vi "myRIO_BRig_Host_v0,20.vi"() -> ()   [LabVIEW 2014]
panel:
  out "output_iTrial":i32
  out "BlockL_T2R_cur":u16 caption="Trials2Reward"
  out "BlockL_BTPR_cur":u16 caption="BadTrialsPostReward"
  out "BlockL_T2R_avg":dbl caption="Trials2Reward" format="%#_3g"
  out "BlockL_BTPR_avg":dbl caption="BadTrialsPostReward" format="%#_3g"
  out "BlockR_T2R_cur":u16 caption="Trials2Reward"
  out "BlockR_BTPR_cur":u16 caption="BadTrialsPostReward"
  out "BlockR_T2R_avg":dbl caption="Trials2Reward" format="%#_3g"
  out "BlockR_BTPR_avg":dbl caption="BadTrialsPostReward" format="%#_3g"
  out "RunTime_minutes":u16
  out "RunTime_seconds":u16
  out "error out 2":errorcluster caption="error out"
  in  "dataIn_maxTrialsDisplayed":u16 caption="Number of Trials Displayed\n( 0 = all trials )"
  in  "colorIn_timeout":u32(colorbox)=7468543 caption="Choice Timeout"
  in  "colorIn_wrong/cue":u32(colorbox)=16728618 caption="Wrong Choice or\nLicked During Cue"
  in  "colorIn_reward":u32(colorbox)=5898088 caption="Reward"
  in  "colorIn_unknown":u32(colorbox)=16449331 caption="Unknown Trial Status"
  in  "LoadPrevSettings":bool
  out "dataOut_plot":cluster{i32[], i32[]}[](graph)
  out "iBlock":u16
  out "iTrial":u16
  in  "stop":bool
  # "Exp Stats"
  # "Current Block Stats"
  # "Trials 2 Reward\n\nBad Trials\nPost Reward"
  # "Left Spout    Right Spout"
  # "Run Time\n\n   minutes    seconds"
  # "Average Block Stats"
  # "Trials 2 Reward\n\nBad Trials\nPost Reward"
  # "Left Spout    Right Spout"
  # "If you get ERROR 5 related to opening a file, press CONTINUE"
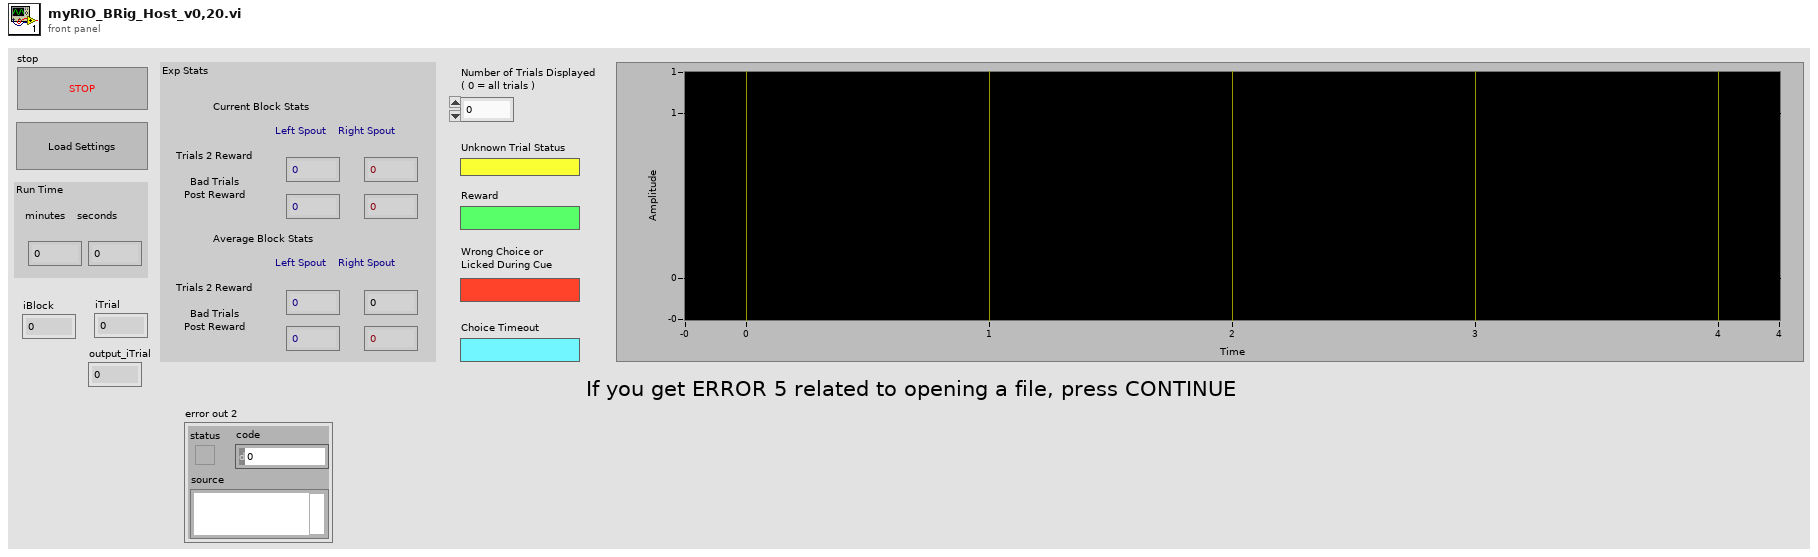
[diagram p1: front panel]
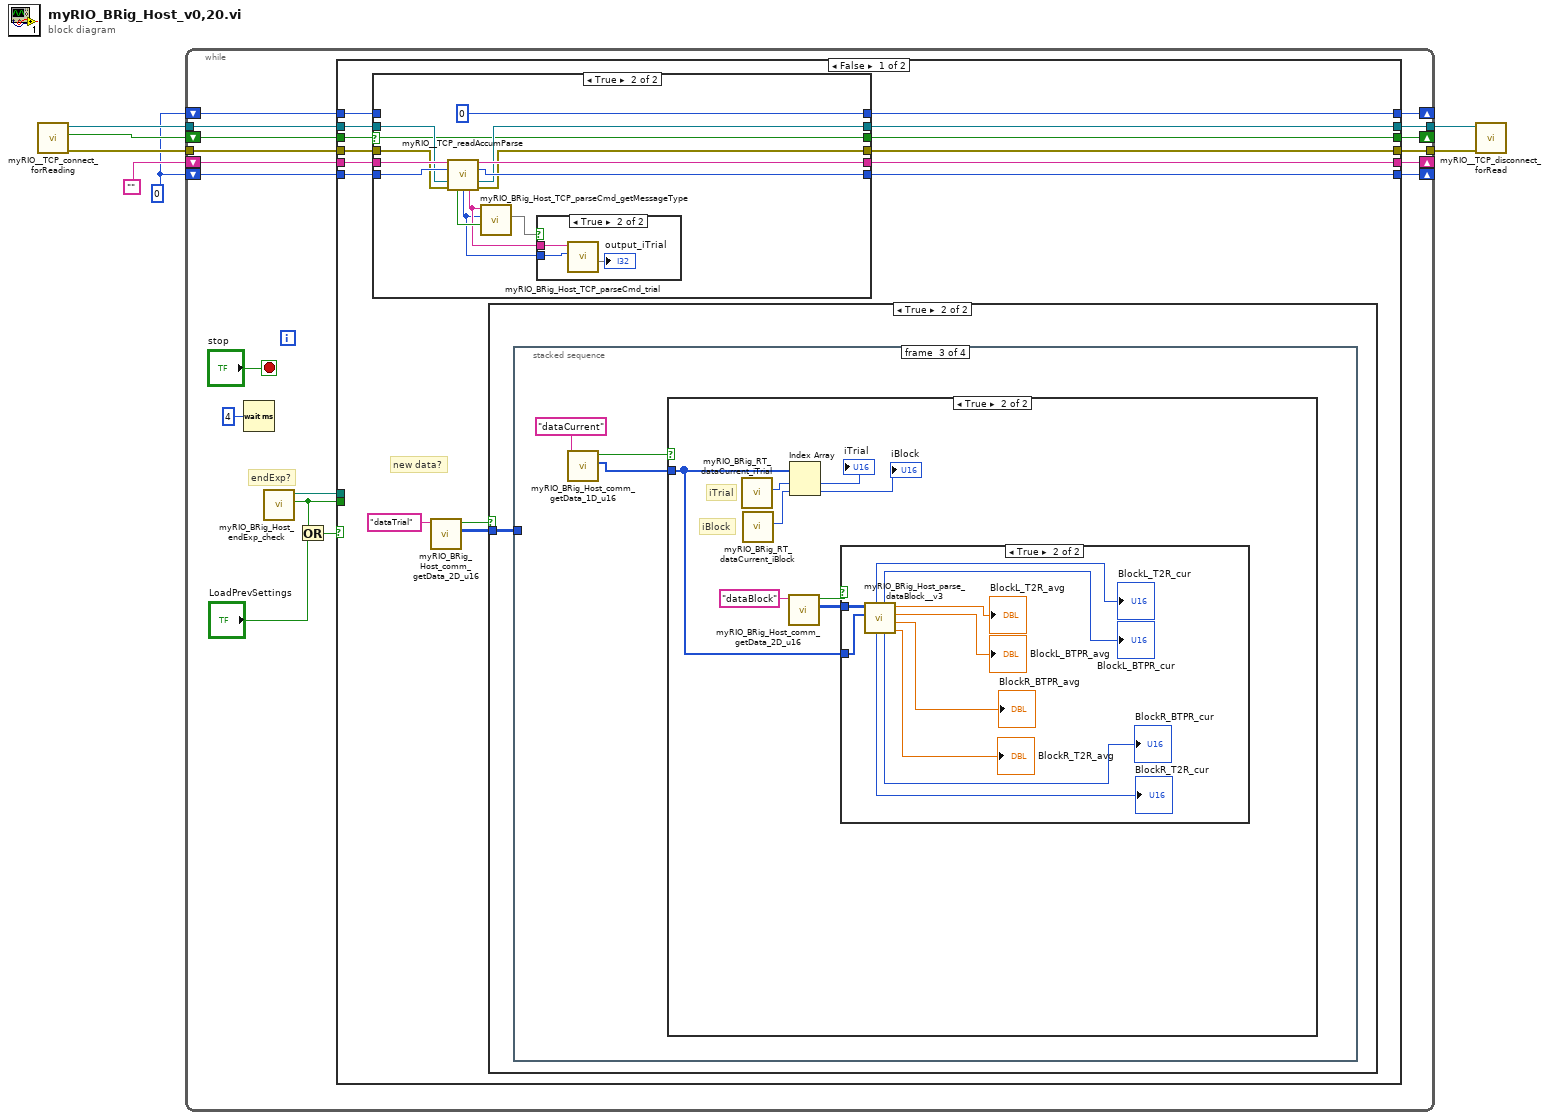
[diagram p0: block diagram]
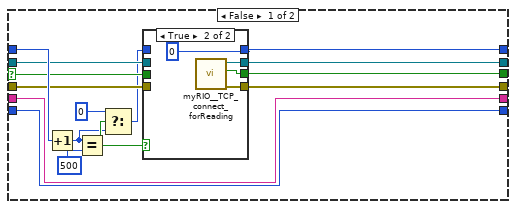
[diagram p2: hidden frame]
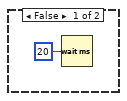
[diagram p5: hidden frame]
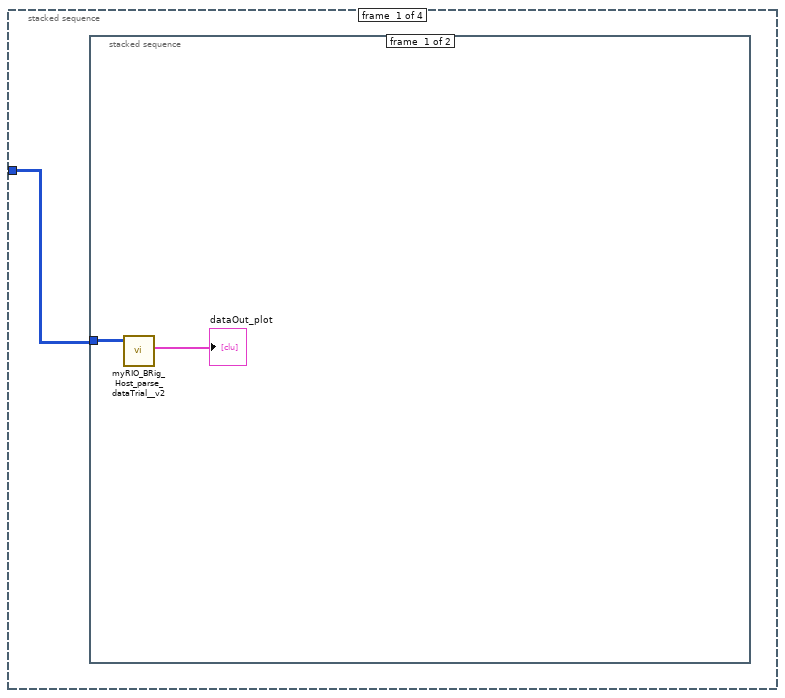
[diagram p6: hidden frame]
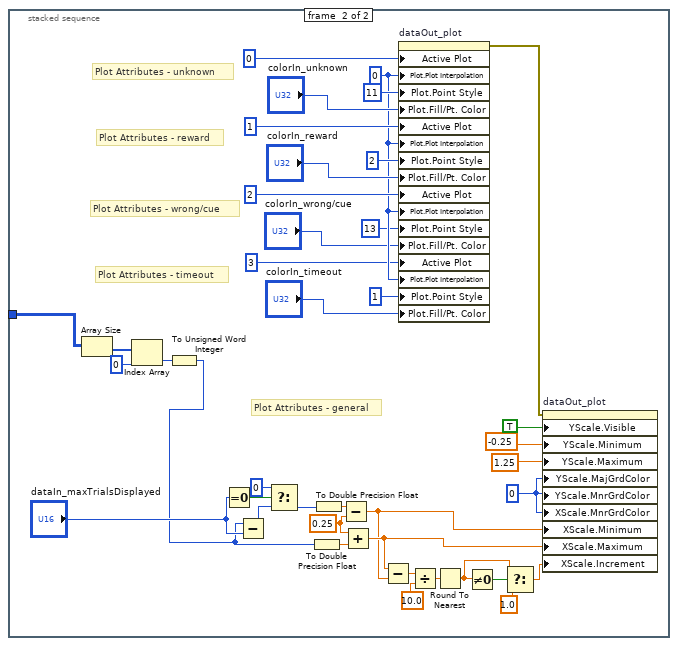
[diagram p7: hidden frame]
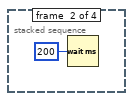
[diagram p8: hidden frame]
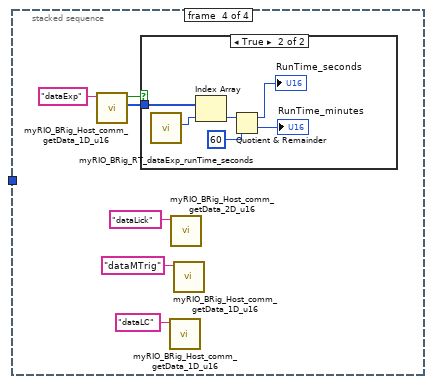
[diagram p11: hidden frame]
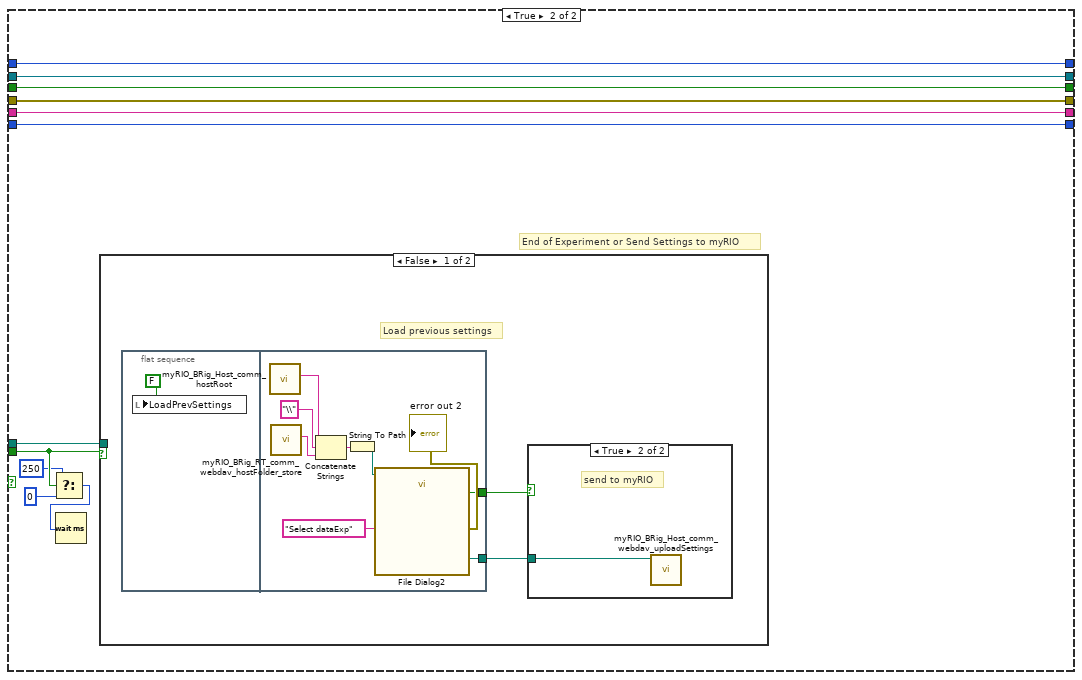
[diagram p13: hidden frame]
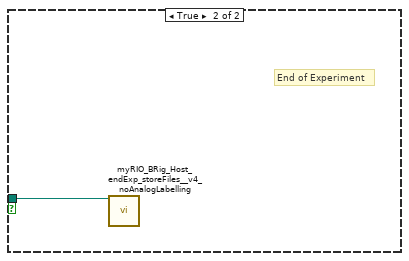
[diagram p15: hidden frame]
diagram:
  w1 = 0
  n1 = call "myRIO__TCP_connect_forReading.vi"() -> ("output_error"=w6:errorcluster, "output_connected"=w5:bool, "output_hTCP"=w7:refnum<k5>)  [unwired: 9 in]
  n2 = while {
    tunnel: w7 -> [w19]
    tunnel: w6 -> [w17]
    tunnel: [w18] -> w4
    tunnel: [w16] -> w3
    shift-right: [w13] -> _
    shift-left: "" -> [w15]
    shift-right: [w12] -> _
    shift-left: w1 -> [w14]
    shift-right: [w10] -> _
    shift-left: w5 -> [w11]
    shift-right: [w8] -> _
    shift-left: w1 -> [w9]
    stop <- "stop" stop-if-true
    # "endExp?"
    n3 = Wait (ms)(milliseconds to wait=u32 4) -> ()  [unwired: 1 out]
    n4 = call "myRIO_BRig_Host_endExp_check.vi"() -> ("output_IendExp"=w23:bool, "output_filePath_expExp"=w22:path)  [unwired: 10 in]
    n5 = Or(x=w23, y="LoadPrevSettings") -> (x .or. y?=w24:bool)
    n6 = case shown="False" w24 {
      tunnel: w23 -> [_ w169]
      tunnel: w22 -> [_ w170]
      tunnel: w19 -> [w33 w165]
      tunnel: [w32 w165] -> w18
      tunnel: w17 -> [w31 w164]
      tunnel: [w30 w164] -> w16
      tunnel: w15 -> [w37 w163]
      tunnel: w14 -> [w36 w162]
      tunnel: [w35 w163] -> w13
      tunnel: [w34 w162] -> w12
      tunnel: w11 -> [w29 w161]
      tunnel: [w28 w161] -> w10
      tunnel: w9 -> [w27 w160]
      tunnel: [w26 w160] -> w8
      frame False {
        # "new data?"
        n7 = case shown="True" w29 {
          selector: w29 -> [w48 w69]
          tunnel: w37 -> [w41 w77]
          tunnel: w36 -> [w42 w76]
          tunnel: [w41 w75] -> w35
          tunnel: [w42 w74] -> w34
          tunnel: w33 -> [w49 w73]
          tunnel: [w52 w72] -> w32
          tunnel: w31 -> [w47 w71]
          tunnel: [w51 w70] -> w30
          tunnel: [w50 w69] -> w28
          tunnel: w27 -> [w54 _]
          tunnel: [w53 0] -> w26
          frame False {
            n8 = Increment(x=w54) -> (x+1=w45:i32)
            n9 = Equal?(x=w45, y=500) -> (x = y?=w46:bool)
            n10 = Select(t=0, s=w46, f=w45) -> (s? t:f=w43:i32)
            n11 = case shown="True" w46 {
              tunnel: w43 -> [w59 _]
              tunnel: [w59 0] -> w53
              tunnel: [w58 w62] -> w52
              tunnel: [w56 w61] -> w51
              tunnel: [w57 w60] -> w50
              tunnel: w49 -> [w58 _]
              tunnel: w48 -> [w57 _]
              tunnel: w47 -> [w56 _]
              frame False {
              }
              frame True {
                n12 = call "myRIO__TCP_connect_forReading.vi"() -> ("output_error"=w61:errorcluster, "output_connected"=w60:bool, "output_hTCP"=w62:refnum<k5>)  [unwired: 9 in]
              }
            }
          }
          frame True {
            n13 = call "myRIO__TCP_readAccumParse.vi"("input_strAccum"=w77, "input_count"=w76, "input_handle_TCP"=w73, "input_error"=w71) -> ("output_strAccum"=w75:string, "output_count"=w74:i32, "output_handle_TCP"=w72:refnum<k5>, "output_haveCmd"=w67:bool, "output_countCmd"=w64:i32, "output_strCmd"=w65:string, "output_error"=w70:errorcluster)  [unwired: 5 in]
            n14 = call "myRIO_BRig_Host_TCP_parseCmd_getMessageType.vi"("input_haveCmd"=w67, "input_countCmd"=w64, "input_strCmd"=w65) -> (2:w66)  [unwired: 7 in, 1 out]
            n15 = case shown="True" w66 {
              tunnel: w65 -> [_ w80]
              tunnel: w64 -> [_ w79]
              frame False {
              }
              frame True {
                n16 = call "myRIO_BRig_Host_TCP_parseCmd_trial.vi"("input_countCmd"=w79, "input_strCmd"=w80) -> (1:→"output_iTrial")  [unwired: 7 in, 2 out]
              }
            }
          }
        }
        n17 = call "myRIO_BRig_Host_comm_getData_2D_u16.vi"("input_fileName"="dataTrial") -> ("output_data_2D"=w38:u16[][], "output_I_data"=w39:bool)  [unwired: 9 in]
        n18 = case shown="True" w39 {
          tunnel: w38 -> [_ w82]
          frame False {
            n19 = Wait (ms)(milliseconds to wait=u32 20) -> ()  [unwired: 1 out]
          }
          frame True {
            n20 = stacked-sequence {
              tunnel: w82 -> [w83 _ _ _]
              frame #0 {
                n21 = stacked-sequence {
                  tunnel: w83 -> [w84 w90]
                  frame #0 {
                    n22 = call "myRIO_BRig_Host_parse_dataTrial__v2.vi"("arrayIn_dataTrial"=w84) -> ("appended array"=→"dataOut_plot":cluster{i32[], i32[]}[])  [unwired: 10 in]
                  }
                  frame #1 {
                    w105 = 0.25 ("y")
                    w109 = u32 0 ("Y Scale.Grid Colors:Major Color")
                    w118 = u8 0 ("Plot.Plot Interpolation")
                    # "Plot Attributes - general"
                    # "Plot Attributes - timeout"
                    # "Plot Attributes - wrong/cue"
                    # "Plot Attributes - reward"
                    # "Plot Attributes - unknown"
                    n23 = Array Size(array=w90) -> (size(s)=w92:i32[])
                    n24 = Index Array(array=w92, index=0) -> (element=w88:i32)
                    n25 = To Unsigned Word Integer(number=w88) -> (unsigned 16bit integer=w87:u16)
                    n26 = Equal To 0?(x="dataIn_maxTrialsDisplayed") -> (x = 0?=w108:bool)
                    n27 = Subtract(x=w87, y="dataIn_maxTrialsDisplayed") -> (x-y=w107:u16)
                    n28 = Select(t=u16 0, s=w108, f=w107) -> (s? t:f=w102:u16)
                    n29 = To Double Precision Float(number=w87) -> (double precision float=w104:dbl)
                    n30 = To Double Precision Float(number=w102) -> (double precision float=w103:dbl)
                    n31 = Subtract(x=w103, y=w105) -> (x-y=w94:dbl)
                    n32 = Add(x=w105, y=w104) -> (x+y=w95:dbl)
                    n33 = Subtract(x=w95, y=w94) -> (x-y=w101:dbl)
                    n34 = property on="dataOut_plot" class="XYGraph (strict)"("Active Plot"=u32 0, "Plot.Plot Interpolation"=w118, "Plot.Point Style"=u8 11, "Plot.Fill/Pt. Color"="colorIn_unknown", "Active Plot"=u32 1, "Plot.Plot Interpolation"=w118, "Plot.Point Style"=u8 2, "Plot.Fill/Pt. Color"="colorIn_reward", "Active Plot"=u32 2, "Plot.Plot Interpolation"=w118, "Plot.Point Style"=u8 13, "Plot.Fill/Pt. Color"="colorIn_wrong/cue", "Active Plot"=u32 3, "Plot.Plot Interpolation"=w118, "Plot.Point Style"=u8 1, "Plot.Fill/Pt. Color"="colorIn_timeout") -> (error out=w93:errorcluster)  [unwired: 2 in, 1 out]
                    n35 = Divide(x=w101, y=10.0) -> (x/y=w99:dbl)
                    n36 = Round To Nearest(number=w99) -> (nearest integer value=w97:dbl)
                    n37 = Not Equal To 0?(x=w97) -> (x != 0?=w98:bool)
                    n38 = Select(t=w97, s=w98, f=1.0) -> (s? t:f=w96:dbl)
                    n39 = property on="dataOut_plot" class="XYGraph (strict)"(error in=w93, "YScale.Visible"=TRUE ("Y Scale.Visible"), "YScale.Minimum"=-0.25 ("Y Scale.Range:Minimum"), "YScale.Maximum"=1.25 ("Y Scale.Range:Maximum"), "YScale.MajGrdColor"=w109, "YScale.MnrGrdColor"=w109, "XScale.MnrGrdColor"=w109, "XScale.Minimum"=w94, "XScale.Maximum"=w95, "XScale.Increment"=w96) -> ()  [unwired: 1 in, 2 out]
                  }
                }
              }
              frame #1 {
                n40 = Wait (ms)(milliseconds to wait=u32 200) -> ()  [unwired: 1 out]
              }
              frame #2 {
                n41 = call "myRIO_BRig_Host_comm_getData_1D_u16.vi"("input_fileName"="dataCurrent") -> ("output_data_1D"=w127:u16[], "output_I_data"=w128:bool)  [unwired: 9 in]
                n42 = case shown="True" w128 {
                  tunnel: w127 -> [_ w130]
                  frame False {
                  }
                  frame True {
                    # "iBlock"
                    # "iTrial"
                    n43 = call "myRIO_BRig_RT_dataCurrent_iTrial.vi"() -> ("output_iTrial"=w137:i32)  [unwired: 11 in]
                    n44 = call "myRIO_BRig_RT_dataCurrent_iBlock.vi"() -> ("output_iBlock"=w136:i32)  [unwired: 11 in]
                    n45 = call "myRIO_BRig_Host_comm_getData_2D_u16.vi"("input_fileName"="dataBlock") -> ("output_data_2D"=w131:u16[][], "output_I_data"=w132:bool)  [unwired: 9 in]
                    n46 = Index Array(array=w130, index #1=w137, index #2=w136) -> (element #1=→"iTrial":u16, element #2=→"iBlock":u16)
                    n47 = case shown="True" w132 {
                      tunnel: w131 -> [_ w139]
                      tunnel: w130 -> [_ w138]
                      frame False {
                      }
                      frame True {
                        n48 = call "myRIO_BRig_Host_parse_dataBlock__v3.vi"("input_dataCurrent"=w138, "input_dataBlock"=w139) -> ("BlockR_T2R_avg"=→"BlockR_T2R_avg":dbl, "BlockR_BTPR_avg"=→"BlockR_BTPR_avg":dbl, "BlockL_BTPR_avg"=→"BlockL_BTPR_avg":dbl, "BlockL_T2R_avg"=→"BlockL_T2R_avg":dbl, "BlockR_BTPR_cur"=→"BlockR_BTPR_cur":u16, "BlockL_BTPR_cur"=→"BlockL_BTPR_cur":u16, "BlockR_T2R_cur"=→"BlockR_T2R_cur":u16, "BlockL_T2R_cur"=→"BlockL_T2R_cur":u16)  [unwired: 2 in]
                      }
                    }
                  }
                }
              }
              frame #3 {
                n49 = call "myRIO_BRig_Host_comm_getData_1D_u16.vi"("input_fileName"="dataExp") -> ("output_data_1D"=w151:u16[], "output_I_data"=w152:bool)  [unwired: 9 in]
                n50 = case shown="True" w152 {
                  tunnel: w151 -> [_ w159]
                  frame False {
                  }
                  frame True {
                    n51 = call "myRIO_BRig_RT_dataExp_runTime_seconds.vi"() -> ("output_RunTime_minutes"=w158:i32)  [unwired: 11 in]
                    n52 = Index Array(array=w159, index=w158) -> (element=w157:u16)
                    n53 = Quotient & Remainder(x=w157, y=u16 60) -> (x-y*floor(x/y)=→"RunTime_seconds":u16, floor(x/y)=→"RunTime_minutes":u16)
                  }
                }
                n54 = call "myRIO_BRig_Host_comm_getData_1D_u16.vi"("input_fileName"="dataLC") -> ()  [unwired: 9 in, 2 out]
                n55 = call "myRIO_BRig_Host_comm_getData_2D_u16.vi"("input_fileName"="dataLick") -> ()  [unwired: 9 in, 2 out]
                n56 = call "myRIO_BRig_Host_comm_getData_1D_u16.vi"("input_fileName"="dataMTrig") -> ()  [unwired: 9 in, 2 out]
              }
            }
          }
        }
      }
      frame True {
        # "End of Experiment or Send Settings to myRIO"
        n57 = Select(t=u32 250 ("milliseconds to wait"), s=w169, f=u32 0 ("milliseconds to wait")) -> (s? t:f=w167:u32)
        n58 = Wait (ms)(milliseconds to wait=w167) -> ()  [unwired: 1 out]
        n59 = case shown="False" w169 {
          tunnel: w170 -> [_ w184]
          frame False {
            # "Load previous settings"
            n60 = flat-sequence {
              tunnel: [w176] -> w171
              tunnel: [w175] -> w172
              frame #0 {
                n61 = local write "LoadPrevSettings"(FALSE ("LoadPrevSettings")) -> ()
              }
              frame #1 {
                n62 = call "myRIO_BRig_Host_comm_hostRoot.vi"() -> ("output_hostRoot"=w178:string)  [unwired: 11 in]
                n63 = call "myRIO_BRig_RT_comm_webdav_hostFolder_store.vi"() -> ("output_HostFolder"=w180:string)  [unwired: 11 in]
                n64 = Concatenate Strings(w178, "\\" ("string"), w180) -> (w182:string)
                n65 = String To Path(string=w182) -> (path=w181:path)
                n66 = call "File Dialog2"("start path"=w181, "prompt"="Select dataExp") -> ("selected path"=w176:path, "exists"=w175:bool, "error out"=→"error out 2":errorcluster)  [unwired: 10 in, 1 out]
              }
            }
            n67 = case shown="True" w172 {
              tunnel: w171 -> [_ w173]
              frame False {
                # "invalid file\nor\ncancelled"
              }
              frame True {
                # "send to myRIO"
                n68 = call "myRIO_BRig_Host_comm_webdav_uploadSettings.vi"("input_filePath"=w173) -> ()  [unwired: 11 in]
              }
            }
          }
          frame True {
            # "End of Experiment"
            n69 = call "myRIO_BRig_Host_endExp_storeFiles__v4_noAnalogLabelling.vi"("input_filePath"=w184) -> ()  [unwired: 15 in]
          }
        }
      }
    }
  }
  n70 = call "myRIO__TCP_disconnect_forRead.vi"("input_error"=w3, "input_hTCP"=w4) -> ()  [unwired: 9 in, 1 out]
